vi "Final_Cluster_Key.vi"(7 "AllObjs[]":refnum<vi>[](array[refnum]), 8 "error in (no error)":errorcluster, 9 "Label.Text":string, 10 "String":string, 11 "Refnum in":T1) -> (0 "error out":errorcluster, 3 "Refnum out":T1)   [LabVIEW 2014]
uses:
  <vilib>/Utility/config.llb/Config Data RefNum.ctl
  <vilib>/Utility/config.llb/Read Key (Double).vi
  <vilib>/Utility/config.llb/Read Key (String).vi
  <vilib>/Utility/config.llb/Read Key (Path).vi
  <vilib>/Utility/config.llb/Read Key (I32).vi
  <vilib>/Utility/config.llb/Read Key (U32).vi
  <vilib>/Utility/config.llb/Read Key (Boolean).vi
  <vilib>/Utility/config.llb/NI_LVConfig.lvlib
  <vilib>/Utility/VariantDataType/VariantType.lvlib
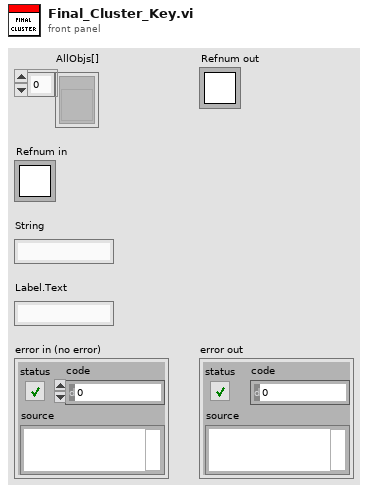
[diagram p1: front panel]
types:
  T1 = typedef "NI_LVConfig.lvlib/Config Data RefNum.ctl" = refnum<k1>
  T2 = typedef "VariantType.lvlib/Type.ctl" = enum8{"Invalid Type", "Void", "I8", "I16", "I32", "I64", "U8", "U16", "U32", "U64", "Single Float", "Double Float", "Extended Float", "Single Complex", "Double Complex", "Extended Complex", "Enum U8", "Enum U16", "Enum U32", "Enum U64", "Single Float With Unit", "Double Float With Unit", "Extended Float With Unit", "Single Complex with Unit", "Double Complex with Unit", "Extended Complex with Unit", "Boolean", "String", "Path", "Picture", "Tag", "Array", "Cluster", "Variant", "LV Variant", "Waveform", "Timestamp", "Digital Waveform", "Digital Data", "ExpressData", "Refnum", "External Data", "VI", "Poly VI", "LabVIEW Class Instance", "Fixed Point"}
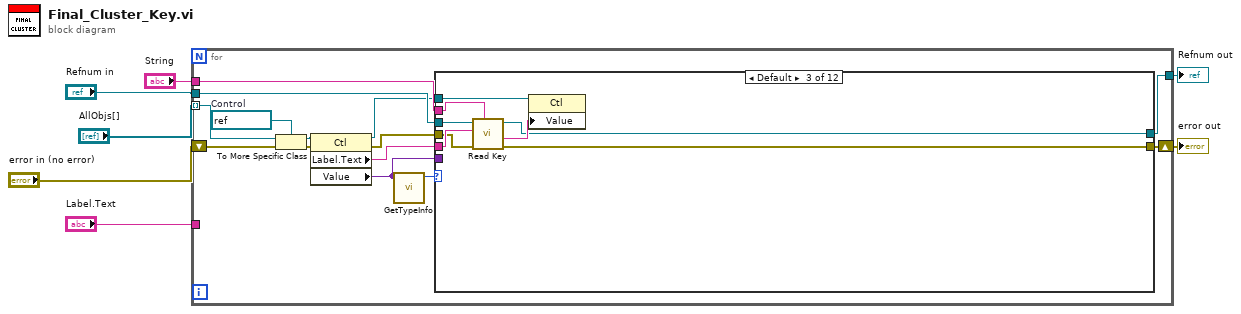
[diagram p0: block diagram]
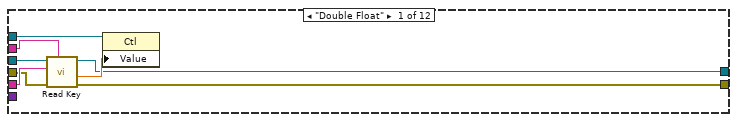
[diagram p2: hidden frame]
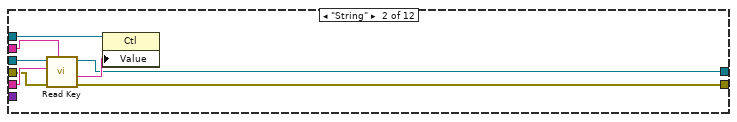
[diagram p3: hidden frame]
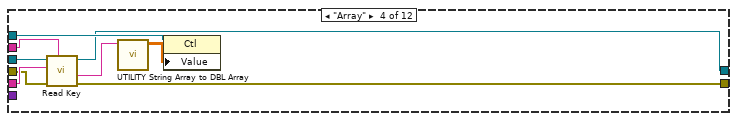
[diagram p4: hidden frame]
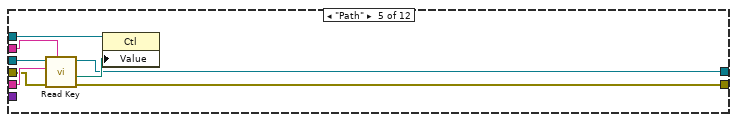
[diagram p5: hidden frame]
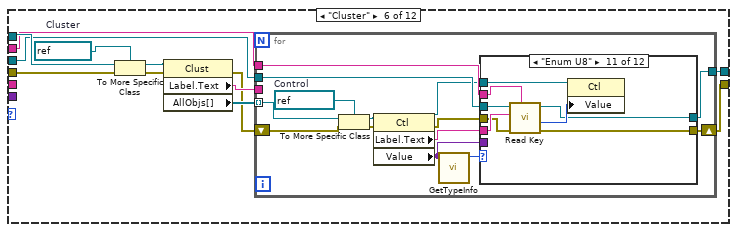
[diagram p6: hidden frame]
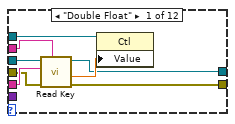
[diagram p7: hidden frame]
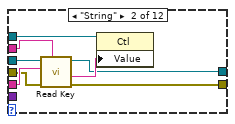
[diagram p8: hidden frame]
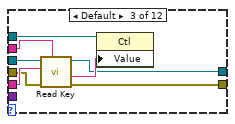
[diagram p9: hidden frame]
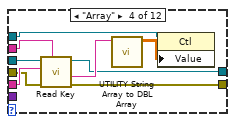
[diagram p10: hidden frame]
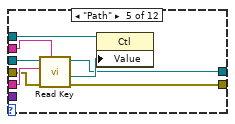
[diagram p11: hidden frame]
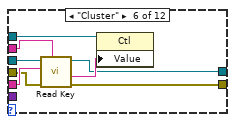
[diagram p12: hidden frame]
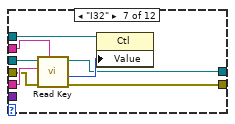
[diagram p13: hidden frame]
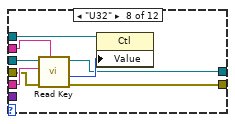
[diagram p14: hidden frame]
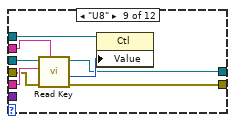
[diagram p15: hidden frame]
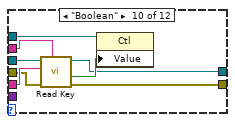
[diagram p16: hidden frame]
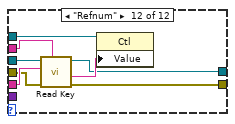
[diagram p17: hidden frame]
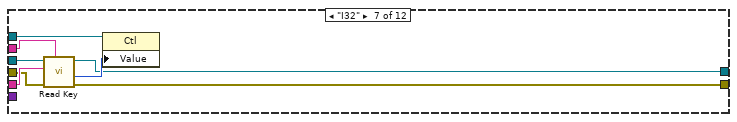
[diagram p18: hidden frame]
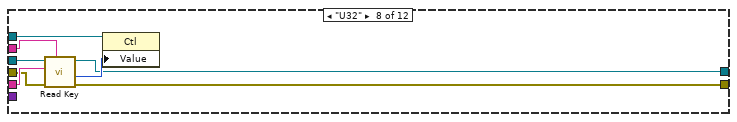
[diagram p19: hidden frame]
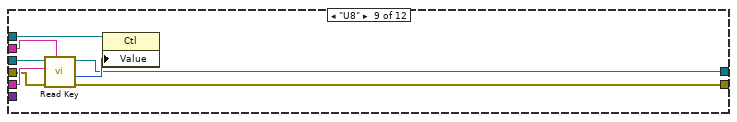
[diagram p20: hidden frame]
diagram:
  n1 = for {
    tunnel: "String" -> [w21]
    tunnel: [w20] -> w1
    tunnel: "Refnum in" -> [w16]
    tunnel: "AllObjs[]" -> [w12] mode=indexing
    tunnel: "Label.Text" -> [_]
    shift-right: [w19] -> w2
    shift-left: "error in (no error)" -> [w10]
    w18 = refnum<vi> refnum  # Control
    n2 = To More Specific Class(target class=w18, reference=w12, error in=w10) -> (specific class reference=w17:refnum<vi>, error out=w9:errorcluster)
    n3 = property class="Ctl"(reference=w17, error in=w9) -> (reference out=w11:refnum<vi>, error out=w8:errorcluster, "Label.Text"=w13:string, "Value"=w14:variant)
    n4 = call <vilib>:"GetTypeInfo.vi"("Variant"=w14) -> ("Type Enum"=w15:T2)  [unwired: 6 in, 4 out]
    n5 = case shown="Default" w15 {
      tunnel: w21 -> [w28 w36 w44 w52 w61 w67 w192 w200 w208 w216 w224 w232]
      tunnel: w13 -> [w27 w35 w43 w50 w60 _ w191 w198 w206 w215 w222 w231]
      tunnel: w14 -> [_ _ _ _ _ _ _ _ _ _ _ _]
      tunnel: w16 -> [w26 w34 w42 w51 w59 w66 w190 w199 w207 w213 w223 w230]
      tunnel: [w23 w31 w39 w47 w56 w73 w187 w195 w203 w211 w219 w227] -> w19
      tunnel: [w24 w32 w40 w48 w57 w74 w188 w196 w204 w212 w220 w228] -> w20
      tunnel: w11 -> [w25 w33 w41 w49 w58 w70 w189 w197 w205 w214 w221 w229]
      tunnel: w8 -> [w22 w30 w38 w46 w55 w65 w186 w194 w202 w210 w218 w226]
      frame "Double Float" {
        n6 = call-poly <vilib>:"Read Key.vi"("section"=w28, "error in (no error)"=w22, "key"=w27, "refnum"=w26) -> ("error out"=w23:errorcluster, "value"=w29:dbl, "refnum out"=w24:T1)  [unwired: 4 in, 1 out]
        n7 = property class="Ctl"(reference=w25, "Value"=w29) -> ()  [unwired: 1 in, 2 out]
      }
      frame "String" {
        n8 = call-poly <vilib>:"Read Key.vi"("section"=w36, "error in (no error)"=w30, "key"=w35, "refnum"=w34) -> ("error out"=w31:errorcluster, "value"=w37:string, "refnum out"=w32:T1)  [unwired: 4 in, 1 out]
        n9 = property class="Ctl"(reference=w33, "Value"=w37) -> ()  [unwired: 1 in, 2 out]
      }
      frame Default {
        n10 = call-poly <vilib>:"Read Key.vi"("section"=w44, "error in (no error)"=w38, "key"=w43, "refnum"=w42) -> ("error out"=w39:errorcluster, "value"=w45:string, "refnum out"=w40:T1)  [unwired: 4 in, 1 out]
        n11 = property class="Ctl"(reference=w41, "Value"=w45) -> ()  [unwired: 1 in, 2 out]
      }
      frame "Array" {
        n12 = call-poly <vilib>:"Read Key.vi"("section"=w52, "error in (no error)"=w46, "key"=w50, "refnum"=w51) -> ("error out"=w47:errorcluster, "value"=w53:string, "refnum out"=w48:T1)  [unwired: 4 in, 1 out]
        n13 = call "UTILITY String Array to DBL Array.vi"("String array in"=w53) -> ("Double array out"=w54:dbl[][])  [unwired: 9 in, 1 out]
        n14 = property class="Ctl"(reference=w49, "Value"=w54) -> ()  [unwired: 1 in, 2 out]
      }
      frame "Path" {
        n15 = call-poly <vilib>:"Read Key.vi"("section"=w61, "error in (no error)"=w55, "key"=w60, "refnum"=w59) -> ("error out"=w56:errorcluster, "value"=w62:path, "refnum out"=w57:T1)  [unwired: 4 in, 1 out]
        n16 = property class="Ctl"(reference=w58, "Value"=w62) -> ()  [unwired: 1 in, 2 out]
      }
      frame "Cluster" {
        w71 = refnum<vi> refnum  # Cluster
        n17 = To More Specific Class(target class=w71, reference=w70, error in=w65) -> (specific class reference=w72:refnum<vi>, error out=w64:errorcluster)
        n18 = property class="Clust"(reference=w72, error in=w64) -> (error out=w63:errorcluster, "Label.Text"=w69:string, "AllObjs[]"=w68:refnum<vi>[])  [unwired: 1 out]
        n19 = for {
          tunnel: w67 -> [w88]
          tunnel: [w87] -> w74
          tunnel: w66 -> [w83]
          tunnel: w68 -> [w79] mode=indexing
          tunnel: w69 -> [_]
          shift-right: [w86] -> w73
          shift-left: w63 -> [w77]
          w85 = refnum<vi> refnum  # Control
          n20 = To More Specific Class(target class=w85, reference=w79, error in=w77) -> (specific class reference=w84:refnum<vi>, error out=w76:errorcluster)
          n21 = property class="Ctl"(reference=w84, error in=w76) -> (reference out=w78:refnum<vi>, error out=w75:errorcluster, "Label.Text"=w80:string, "Value"=w81:variant)
          n22 = call <vilib>:"GetTypeInfo.vi"("Variant"=w81) -> ("Type Enum"=w82:T2)  [unwired: 6 in, 4 out]
          n23 = case shown="\"Enum U8\"" w82 {
            tunnel: w88 -> [w95 w101 w111 w119 w127 w133 w142 w152 w157 w168 w176 w181]
            tunnel: w80 -> [w94 w100 w110 w117 w126 w132 w140 w150 w156 w166 w174 w180]
            tunnel: w81 -> [_ _ _ _ _ _ _ _ _ _ _ _]
            tunnel: w83 -> [w92 w102 w109 w118 w128 w134 w141 w151 w158 w167 w175 w182]
            tunnel: [w90 w98 w106 w114 w123 w136 w144 w147 w160 w164 w171 w184] -> w86
            tunnel: [w91 w99 w107 w115 w125 w135 w143 w148 w159 w163 w172 w183] -> w87
            tunnel: w78 -> [w93 w103 w108 w116 w124 w131 w139 w149 w155 w165 w173 w179]
            tunnel: w75 -> [w89 w97 w105 w113 w122 w130 w138 w146 w154 w162 w170 w178]
            frame "Double Float" {
              n24 = call-poly <vilib>:"Read Key.vi"("section"=w95, "error in (no error)"=w89, "key"=w94, "refnum"=w92) -> ("error out"=w90:errorcluster, "value"=w96:dbl, "refnum out"=w91:T1)  [unwired: 4 in, 1 out]
              n25 = property class="Ctl"(reference=w93, "Value"=w96) -> ()  [unwired: 1 in, 2 out]
            }
            frame "String" {
              n26 = call-poly <vilib>:"Read Key.vi"("section"=w101, "error in (no error)"=w97, "key"=w100, "refnum"=w102) -> ("error out"=w98:errorcluster, "value"=w104:string, "refnum out"=w99:T1)  [unwired: 4 in, 1 out]
              n27 = property class="Ctl"(reference=w103, "Value"=w104) -> ()  [unwired: 1 in, 2 out]
            }
            frame Default {
              n28 = call-poly <vilib>:"Read Key.vi"("section"=w111, "error in (no error)"=w105, "key"=w110, "refnum"=w109) -> ("error out"=w106:errorcluster, "value"=w112:string, "refnum out"=w107:T1)  [unwired: 4 in, 1 out]
              n29 = property class="Ctl"(reference=w108, "Value"=w112) -> ()  [unwired: 1 in, 2 out]
            }
            frame "Array" {
              n30 = call-poly <vilib>:"Read Key.vi"("section"=w119, "error in (no error)"=w113, "key"=w117, "refnum"=w118) -> ("error out"=w114:errorcluster, "value"=w120:string, "refnum out"=w115:T1)  [unwired: 4 in, 1 out]
              n31 = call "UTILITY String Array to DBL Array.vi"("String array in"=w120) -> ("Double array out"=w121:dbl[][])  [unwired: 9 in, 1 out]
              n32 = property class="Ctl"(reference=w116, "Value"=w121) -> ()  [unwired: 1 in, 2 out]
            }
            frame "Path" {
              n33 = call-poly <vilib>:"Read Key.vi"("section"=w127, "error in (no error)"=w122, "key"=w126, "refnum"=w128) -> ("error out"=w123:errorcluster, "value"=w129:path, "refnum out"=w125:T1)  [unwired: 4 in, 1 out]
              n34 = property class="Ctl"(reference=w124, "Value"=w129) -> ()  [unwired: 1 in, 2 out]
            }
            frame "Cluster" {
              n35 = call-poly <vilib>:"Read Key.vi"("section"=w133, "error in (no error)"=w130, "key"=w132, "refnum"=w134) -> ("error out"=w136:errorcluster, "value"=w137:string, "refnum out"=w135:T1)  [unwired: 4 in, 1 out]
              n36 = property class="Ctl"(reference=w131, "Value"=w137) -> ()  [unwired: 1 in, 2 out]
            }
            frame "I32" {
              n37 = call-poly <vilib>:"Read Key.vi"("section"=w142, "error in (no error)"=w138, "key"=w140, "refnum"=w141) -> ("error out"=w144:errorcluster, "value"=w145:i32, "refnum out"=w143:T1)  [unwired: 4 in, 1 out]
              n38 = property class="Ctl"(reference=w139, "Value"=w145) -> ()  [unwired: 1 in, 2 out]
            }
            frame "U32" {
              n39 = call-poly <vilib>:"Read Key.vi"("section"=w152, "error in (no error)"=w146, "key"=w150, "refnum"=w151) -> ("error out"=w147:errorcluster, "value"=w153:u32, "refnum out"=w148:T1)  [unwired: 4 in, 1 out]
              n40 = property class="Ctl"(reference=w149, "Value"=w153) -> ()  [unwired: 1 in, 2 out]
            }
            frame "U8" {
              n41 = call-poly <vilib>:"Read Key.vi"("section"=w157, "error in (no error)"=w154, "key"=w156, "refnum"=w158) -> ("error out"=w160:errorcluster, "value"=w161:u32, "refnum out"=w159:T1)  [unwired: 4 in, 1 out]
              n42 = property class="Ctl"(reference=w155, "Value"=w161) -> ()  [unwired: 1 in, 2 out]
            }
            frame "Boolean" {
              n43 = call-poly <vilib>:"Read Key.vi"("section"=w168, "error in (no error)"=w162, "key"=w166, "refnum"=w167) -> ("error out"=w164:errorcluster, "value"=w169:bool, "refnum out"=w163:T1)  [unwired: 4 in, 1 out]
              n44 = property class="Ctl"(reference=w165, "Value"=w169) -> ()  [unwired: 1 in, 2 out]
            }
            frame "Enum U8" {
              n45 = call-poly <vilib>:"Read Key.vi"("section"=w176, "error in (no error)"=w170, "key"=w174, "refnum"=w175) -> ("error out"=w171:errorcluster, "value"=w177:u32, "refnum out"=w172:T1)  [unwired: 4 in, 1 out]
              n46 = property class="Ctl"(reference=w173, "Value"=w177) -> ()  [unwired: 1 in, 2 out]
            }
            frame "Refnum" {
              n47 = call-poly <vilib>:"Read Key.vi"("section"=w181, "error in (no error)"=w178, "key"=w180, "refnum"=w182) -> ("error out"=w184:errorcluster, "value"=w185:string, "refnum out"=w183:T1)  [unwired: 4 in, 1 out]
              n48 = property class="Ctl"(reference=w179, "Value"=w185) -> ()  [unwired: 1 in, 2 out]
            }
          }
        }
      }
      frame "I32" {
        n49 = call-poly <vilib>:"Read Key.vi"("section"=w192, "error in (no error)"=w186, "key"=w191, "refnum"=w190) -> ("error out"=w187:errorcluster, "value"=w193:i32, "refnum out"=w188:T1)  [unwired: 4 in, 1 out]
        n50 = property class="Ctl"(reference=w189, "Value"=w193) -> ()  [unwired: 1 in, 2 out]
      }
      frame "U32" {
        n51 = call-poly <vilib>:"Read Key.vi"("section"=w200, "error in (no error)"=w194, "key"=w198, "refnum"=w199) -> ("error out"=w195:errorcluster, "value"=w201:u32, "refnum out"=w196:T1)  [unwired: 4 in, 1 out]
        n52 = property class="Ctl"(reference=w197, "Value"=w201) -> ()  [unwired: 1 in, 2 out]
      }
      frame "U8" {
        n53 = call-poly <vilib>:"Read Key.vi"("section"=w208, "error in (no error)"=w202, "key"=w206, "refnum"=w207) -> ("error out"=w203:errorcluster, "value"=w209:u32, "refnum out"=w204:T1)  [unwired: 4 in, 1 out]
        n54 = property class="Ctl"(reference=w205, "Value"=w209) -> ()  [unwired: 1 in, 2 out]
      }
      frame "Boolean" {
        n55 = call-poly <vilib>:"Read Key.vi"("section"=w216, "error in (no error)"=w210, "key"=w215, "refnum"=w213) -> ("error out"=w211:errorcluster, "value"=w217:bool, "refnum out"=w212:T1)  [unwired: 4 in, 1 out]
        n56 = property class="Ctl"(reference=w214, "Value"=w217) -> ()  [unwired: 1 in, 2 out]
      }
      frame "Enum U8" {
        n57 = call-poly <vilib>:"Read Key.vi"("section"=w224, "error in (no error)"=w218, "key"=w222, "refnum"=w223) -> ("error out"=w219:errorcluster, "value"=w225:u32, "refnum out"=w220:T1)  [unwired: 4 in, 1 out]
        n58 = property class="Ctl"(reference=w221, "Value"=w225) -> ()  [unwired: 1 in, 2 out]
      }
      frame "Refnum" {
        n59 = call-poly <vilib>:"Read Key.vi"("section"=w232, "error in (no error)"=w226, "key"=w231, "refnum"=w230) -> ("error out"=w227:errorcluster, "value"=w233:string, "refnum out"=w228:T1)  [unwired: 4 in, 1 out]
        n60 = property class="Ctl"(reference=w229, "Value"=w233) -> ()  [unwired: 1 in, 2 out]
      }
    }
  }
  "error out" <- w2
  "Refnum out" <- w1
